vi "save_stabilisation_data.vi"(10 "Stabilisation Data":dbl[][](array[numeric]), 11 "File path for jv data (without scan direction)":path) -> ()   [LabVIEW 2016]
uses:
  <vilib>/Utility/file.llb/Write Delimited Spreadsheet (string).vi
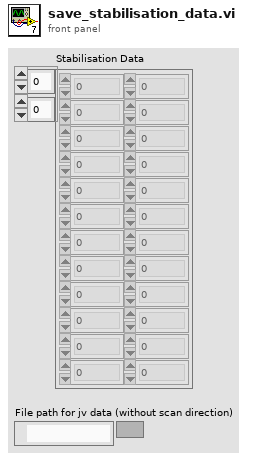
[diagram p1: front panel]
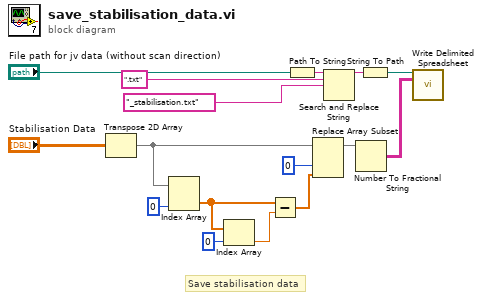
[diagram p0: block diagram]
diagram:
  # "Save stabilisation data"
  n1 = Transpose 2D Array(2D array="Stabilisation Data") -> (transposed array=w12:dbl[][])
  n2 = Index Array(array=w12, index (col)=0 ("disabled index (col)")) -> (element=w10:dbl[])  [unwired: 1 in]
  n3 = Index Array(array=w10, index=0) -> (element=w11:dbl)
  n4 = Subtract(x=w10, y=w11) -> (x-y=w14:dbl[])
  n5 = Path To String(path="File path for jv data (without scan direction)") -> (string=w2:string)
  n6 = Replace Array Subset(array=w12, new element=w14, index (col)=0 ("disabled index (col)")) -> (w15:dbl[][])  [unwired: 1 in]
  n7 = Search and Replace String(input string=w2, search string=".txt", replace string="_stabilisation.txt") -> (result string=w5:string)  [unwired: 5 in, 3 out]
  n8 = Number To Fractional String(number=w15) -> (F-format string=w7:string[][])  [unwired: 3 in]
  n9 = String To Path(string=w5) -> (path=w6:path)
  n10 = call-poly <vilib>:"Write Delimited Spreadsheet.vi"("file path (dialog if empty)"=w6, "2D data"=w7) -> ()  [unwired: 12 in, 2 out]
